vi "act-0020-2-en.vi"() -> ()   [LabVIEW 2010]
uses:
  support/lv_07.lvlib
panel:
  in  "Pu":dbl
  out "Qe":dbl
  in  "Qa":dbl
  out "Cc init":dbl
  out "T init":dbl
  out "Ccpc nv":dbl
  in  "Cc":dbl
  in  "T":dbl
  in  "Ccpc":dbl
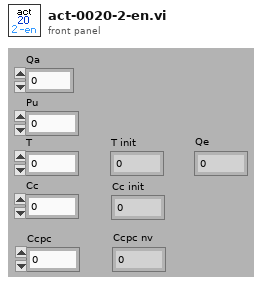
[diagram p1: front panel]
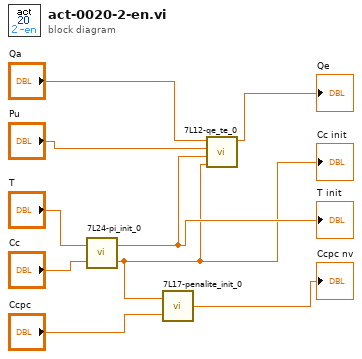
[diagram p0: block diagram]
diagram:
  n1 = call "7L24-pi_init_0.vi"("Cc"="Cc", "T"="T") -> ("Cc init"=w2:dbl, "T init"=w3:dbl)
  "T init" <- w3
  "Cc init" <- w2
  n2 = call "7L17-penalite_init_0.vi"("Ccpc"="Ccpc", "Cc"=w2) -> ("Ccpc init"=→"Ccpc nv":dbl)
  n3 = call "7L12-qe_te_0.vi"("Cc"=w2, "T"=w3, "Pu"="Pu", "Qa"="Qa") -> ("Qe"=→"Qe":dbl)  [unwired: 5 in, 2 out]
